vi "LiftLimit.vi"(11 "PowerIn":dbl) -> (2 "LiftLimit":bool, 3 "PowerOut":dbl)   [LabVIEW 2018]
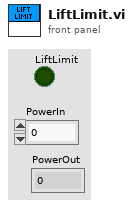
[diagram p1: front panel]
types:
  T1 = typedef "WPI_SwitchDevRef.ctl" = cluster{"DevStatus":errorcluster, "DIO Channel":T2, "CntIndex":T3, "Normally Closed":bool}
  T2 = typedef "FPGA_DIOChannel.ctl" = enum8{"DIO 0", "DIO 1", "DIO 2", "DIO 3", "DIO 4", "DIO 5", "DIO 6", "DIO 7", "DIO 8", "DIO 9", "DIO MXP 0", "DIO MXP 1", "DIO MXP 2", "DIO MXP 3", "DIO MXP 4", "DIO MXP 5", "DIO MXP 6", "DIO MXP 7", "DIO MXP 8", "DIO MXP 9", "DIO MXP 10", "DIO MXP 11", "DIO MXP 12", "DIO MXP 13", "DIO MXP 14", "DIO MXP 15", "SPI Port CS1", "SPI Port CS2", "SPI Port CS3", "SPI Port MISO", "SPI Port MOSI", "Invalid"}
  T3 = typedef "FPGA_CounterCtrSystemIndex.ctl" = enum8{"Ctr 0", "Ctr 1", "Ctr 2", "Ctr 3", "Ctr 4", "Ctr 5", "Ctr 6", "Ctr 7", "Invalid"}
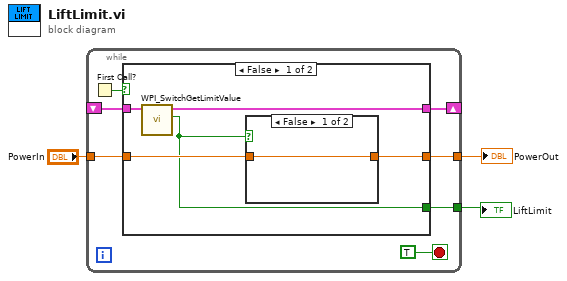
[diagram p0: block diagram]
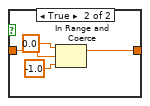
[diagram p2: hidden frame]
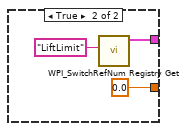
[diagram p3: hidden frame]
diagram:
  n1 = while {
    shift-right: [w8] -> _
    shift-left: _ -> [w7]
    tunnel: "PowerIn" -> [w6]
    tunnel: [w5] -> w1
    tunnel: [w4] -> w3
    stop <- TRUE stop-if-true
    n2 = First Call?() -> (First Call?: T/F=w9:bool)
    n3 = case shown="False" w9 {
      tunnel: [w14 w22] -> w8
      tunnel: w7 -> [w15 _]
      tunnel: w6 -> [w13 _]
      tunnel: [w12 0.0 ("upper limit")] -> w5
      tunnel: [w11 _] -> w4
      frame False {
        n4 = call <vilib>:"WPI_SwitchGetLimitValue.vi"("SwitchDevRef"=w15) -> ("Switch Pressed"=w11:bool, "SwitchDevRef"=w14:T1)  [unwired: 8 in, 1 out]
        n5 = case shown="False" w11 {
          tunnel: w13 -> [w16 w20]
          tunnel: [w16 w17] -> w12
          frame False {
          }
          frame True {
            n6 = In Range and Coerce(upper limit=0.0, x=w20, lower limit=-1.0) -> (coerced(x)=w17:dbl)  [unwired: 1 out]
          }
        }
      }
      frame True {
        n7 = call <vilib>:"WPI_SwitchRefNum Registry Get.vi"("refnum name"="LiftLimit") -> ("SwitchDevRef"=w22:T1)  [unwired: 9 in, 1 out]
      }
    }
  }
  "LiftLimit" <- w3
  "PowerOut" <- w1
